vi "DIAGONAL (SubVI).vi"(0 "9 POSITION CODE":dbl[][](array[numeric])) -> (4 "total":i32, 5 "TL to BR":i32, 6 "TR toBL":i32, 7 "BL to TR":i32, 8 "BR to TL":i32)   [LabVIEW 2009]
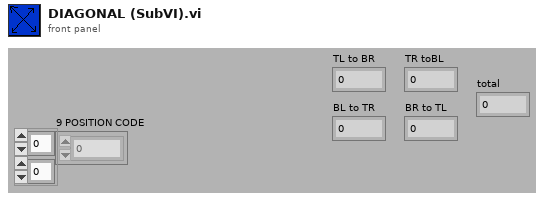
[diagram p1: front panel]
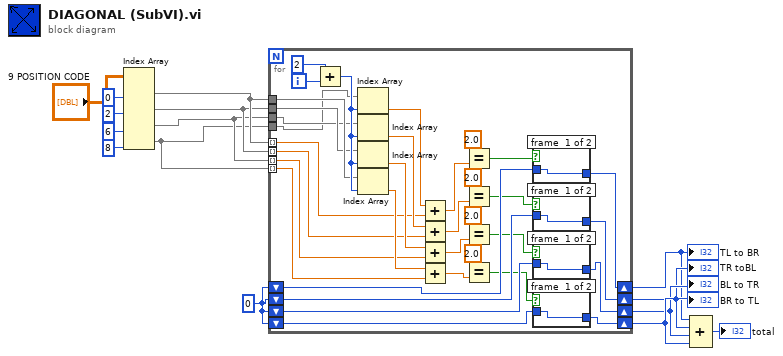
[diagram p0: block diagram]
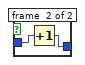
[diagram p2: hidden frame]
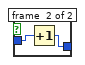
[diagram p3: hidden frame]
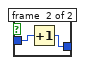
[diagram p4: hidden frame]
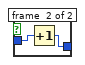
[diagram p5: hidden frame]
diagram:
  w10 = 0 ("disabled index (col)")
  n1 = Index Array(array="9 POSITION CODE", index (col) #1=0 ("disabled index (col)"), index (col) #2=2 ("index (col)"), index (col) #3=6 ("index (col)"), index (col) #4=8 ("index (col)")) -> (element #1=w4:dbl[], element #2=w3:dbl[], element #3=w2:dbl[], element #4=w1:dbl[])  [unwired: 4 in]
  n2 = for {
    tunnel: w4 -> [w19]
    tunnel: w3 -> [w18]
    tunnel: w2 -> [w17]
    tunnel: w1 -> [w16]
    tunnel: w4 -> [w43] mode=indexing
    tunnel: w3 -> [w42] mode=indexing
    tunnel: w2 -> [w41] mode=indexing
    tunnel: w1 -> [w40] mode=indexing
    shift-right: [w33] -> w12
    shift-left: w10 -> [w37]
    shift-right: [w34] -> w13
    shift-left: w10 -> [w38]
    shift-right: [w35] -> w14
    shift-left: w10 -> [w39]
    shift-right: [w32] -> w11
    shift-left: w10 -> [w36]
    i -> [w50]
    n3 = Add(x=2, y=w50) -> (x+y=w48:i32)
    n4 = Index Array(array=w16, index=w48) -> (element=w47:dbl)
    n5 = Index Array(array=w17, index=w48) -> (element=w46:dbl)
    n6 = Index Array(array=w18, index=w48) -> (element=w45:dbl)
    n7 = Index Array(array=w19, index=w48) -> (element=w44:dbl)
    n8 = Add(x=w47, y=w43) -> (x+y=w30:dbl)
    n9 = Add(x=w46, y=w42) -> (x+y=w25:dbl)
    n10 = Add(x=w45, y=w41) -> (x+y=w24:dbl)
    n11 = Add(x=w44, y=w40) -> (x+y=w23:dbl)
    n12 = Equal?(x=2.0, y=w30) -> (x = y?=w29:bool)
    n13 = Equal?(x=2.0, y=w25) -> (x = y?=w22:bool)
    n14 = Equal?(x=2.0, y=w24) -> (x = y?=w21:bool)
    n15 = Equal?(x=2.0, y=w23) -> (x = y?=w20:bool)
    n16 = case shown="True" w29 {
      tunnel: [w51 w53] -> w32
      tunnel: w36 -> [w51 w52]
      frame #0 {
      }
      frame #1 {
        n17 = Increment(x=w52) -> (x+1=w53:i32)
      }
    }
    n18 = case shown="False" w22 {
      tunnel: [w60 w62] -> w33
      tunnel: w37 -> [w60 w61]
      frame #0 {
      }
      frame #1 {
        n19 = Increment(x=w61) -> (x+1=w62:i32)
      }
    }
    n20 = case shown="False" w21 {
      tunnel: [w57 w59] -> w34
      tunnel: w38 -> [w57 w58]
      frame #0 {
      }
      frame #1 {
        n21 = Increment(x=w58) -> (x+1=w59:i32)
      }
    }
    n22 = case shown="False" w20 {
      tunnel: [w54 w56] -> w35
      tunnel: w39 -> [w54 w55]
      frame #0 {
      }
      frame #1 {
        n23 = Increment(x=w55) -> (x+1=w56:i32)
      }
    }
  }
  "TL to BR" <- w11
  "TR toBL" <- w12
  "BL to TR" <- w13
  "BR to TL" <- w14
  n24 = Compound Arithmetic op=ADD(w11, w12, w13, w14) -> (→"total":i32)
